vi "Protocol.Get Simulated Previously Active DTCs.vi"(8 "error in (no error)":errorcluster, 10 "Address":u8, 11 "Simulated Addresses LUT":variant) -> (0 "error out":errorcluster, 1 "DTC Frame":u8[](array[numeric]), 2 "# of Enabled":u8, 3 "Address found":bool)   [LabVIEW 2015, in "J1939 Addon Engine.lvlib"]
uses:
  J1939 Addon Engine.lvlib
  Types/Engine.Node DTC Settings.ctl
  Shared/Types/Monitor Settings.ctl
  Types/Engine.DTC Settings.ctl
  Shared/Types/Compiled Simulated Settings.ctl
  <vilib>/NI Veristand/Custom Device API/Block Data Reference.ctl
  <vilib>/NI Veristand/Custom Device API/Data Reference.ctl
  Types/Engine.DTC FIFOs.ctl
  <vilib>/NI VeriStand/Custom Device API/Custom Device API.lvlib
  Shared/J1939 Addon Shared.lvlib
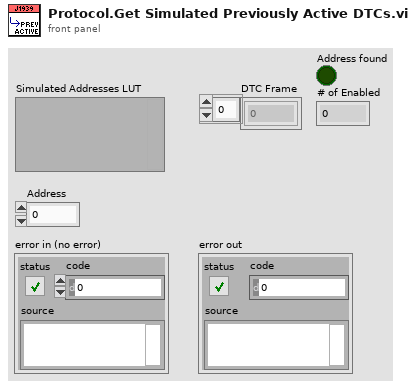
[diagram p1: front panel]
types:
  T1 = typedef "J1939 Addon Engine.lvlib/Engine.Node DTC Settings.ctl" = cluster{"Network":T2, "Sim DTC Refs":T3}
  T2 = typedef "J1939 Addon Shared.lvlib/Monitor Settings.ctl" = cluster{"Address":u8, "Name":u64}
  T3 = typedef "J1939 Addon Engine.lvlib/Engine.DTC Settings.ctl" = cluster{"Data":T4, "FIFOs":T7}
  T4 = typedef "J1939 Addon Shared.lvlib/Compiled Simulated Settings.ctl" = cluster{"DM1 Ref":T5[], "DM1 Value":dbl[], "DM1 Enable Ref":T5[], "DM1 Enable Value":dbl[], "DM2 Ref":T5[], "DM2 Value":dbl[], "DM2 Enable Ref":T5[], "DM2 Enable Value":dbl[]}
  T5 = typedef "Custom Device API.lvlib/Block Data Reference.ctl" = cluster{"Data Reference":T6, "Offset":u64, "Length":u64}
  T6 = typedef "Custom Device API.lvlib/Data Reference.ctl" = i32
  T7 = typedef "J1939 Addon Engine.lvlib/Engine.DTC FIFOs.ctl" = cluster{"DM1 Data":refnum<k33>, "DM1 Enable":refnum<k33>, "DM2 Data":refnum<k33>, "DM2 Enable":refnum<k33>, "DM1 Reset":refnum<k33>, "DM2 Reset":refnum<k33>}
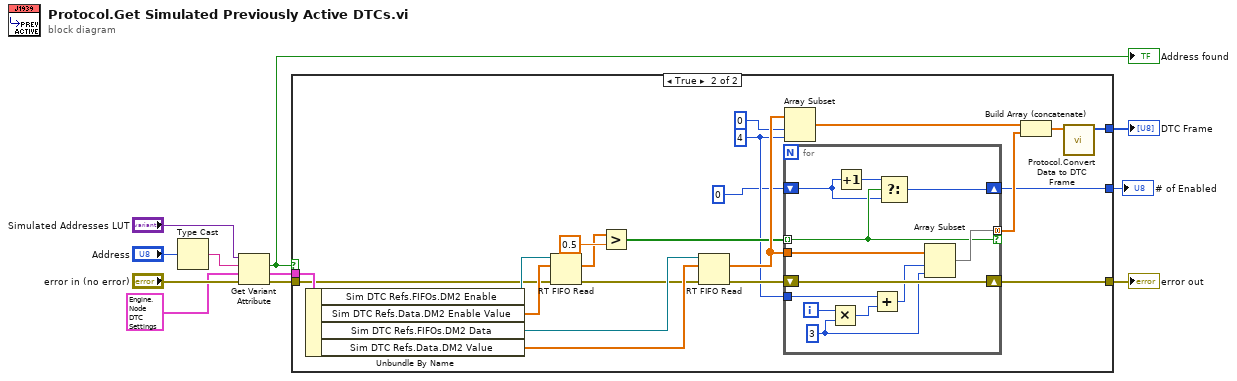
[diagram p0: block diagram]
diagram:
  n1 = Type Cast(x="Address") -> (*(type *) &x=w8:string)  [unwired: 1 in]
  n2 = Get Variant Attribute(Variant="Simulated Addresses LUT", name=w8, default value (empty Variant)=T1 {"Network"={"Address"=0, "Name"=0}, "Sim DTC Refs"={"Data"={"DM1 Ref"=[], "DM1 Value"=[], "DM1 Enable Ref"=[], "DM1 Enable Value"=[], "DM2 Ref"=[], "DM2 Value"=[], "DM2 Enable Ref"=[], "DM2 Enable Value"=[]}, "FIFOs"={"DM1 Data"=refnum, "DM1 Enable"=refnum, "DM2 Data"=refnum, "DM2 Enable"=refnum, "DM1 Reset"=refnum, "DM2 Reset"=refnum}}} ("cluster"), error in="error in (no error)") -> (found=w3:bool, value=w11:T1, error out=w10:errorcluster)  [unwired: 1 out]
  "Address found" <- w3
  n3 = case shown="True" w3 {
    tunnel: w11 -> [_ w26]
    tunnel: w10 -> [w12 w25]
    tunnel: [w12 w23] -> w5
    tunnel: [_ w17] -> w4
    tunnel: [_ w13] -> w2
    frame False {
    }
    frame True {
      w16 = 4 ("length")
      n4 = Unbundle By Name(w26) -> ("Sim DTC Refs.FIFOs.DM2 Enable"=w27:refnum<k33>, "Sim DTC Refs.Data.DM2 Enable Value"=w28:dbl[], "Sim DTC Refs.FIFOs.DM2 Data"=w29:refnum<k33>, "Sim DTC Refs.Data.DM2 Value"=w30:dbl[])
      n5 = RT FIFO Read(0:w27, 1:w28, 3:w25) -> (9:w19:dbl[], 11:w18:errorcluster)  [unwired: 1 in, 3 out]
      n6 = Greater?(x=w19, y=0.5) -> (0:w21:bool[])
      n7 = RT FIFO Read(0:w29, 1:w30, 3:w18) -> (9:w32:dbl[], 11:w22:errorcluster)  [unwired: 1 in, 3 out]
      n8 = for {
        tunnel: w21 -> [w37] mode=indexing
        shift-right: [w45] -> w23
        shift-left: w22 -> [w45]
        tunnel: w32 -> [w44]
        tunnel: [w43] -> w33 mode=concatenating if=w37
        tunnel: w16 -> [w40]
        shift-right: [w36] -> w13
        shift-left: u8 0 -> [w35]
        i -> [w42]
        w38 = 3 ("x")
        n9 = Multiply(x=w42, y=w38) -> (x*y=w41:i32)
        n10 = Increment(x=w35) -> (x+1=w34:u8)
        n11 = Add(x=w40, y=w41) -> (x+y=w39:i32)
        n12 = Select(t=w34, s=w37, f=w35) -> (s? t:f=w36:u8)
        n13 = Array Subset(array=w44, index=w39, length=w38) -> (w43:dbl[])
      }
      n14 = Array Subset(array=w32, index=0, length=w16) -> (w31:dbl[])
      n15 = Build Array (concatenate)(w31, w33) -> (w24:dbl[])
      n16 = call "Protocol.Convert Data to DTC Frame.vi"("Data"=w24) -> ("DTC Frame"=w17:u8[])  [unwired: 10 in]
    }
  }
  "error out" <- w5
  "DTC Frame" <- w4
  "# of Enabled" <- w2
